vi "Get SLSC Module By Slot.vi"(8 "error in (no error)":errorcluster, 10 "Slot":i32, 11 "SLSC Chassis":u64) -> (0 "error out":errorcluster, 2 "SLSC Module":u64, 3 "SLSC Chassis out":u64)   [LabVIEW 2017, in "VeriStand SLSC Scripting.lvlib"]
uses:
  VeriStand SLSC Scripting.lvlib
  NationalInstruments.VeriStand.SystemDefinitionAPI
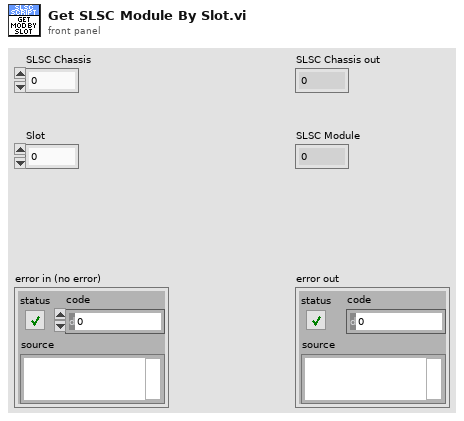
[diagram p1: front panel]
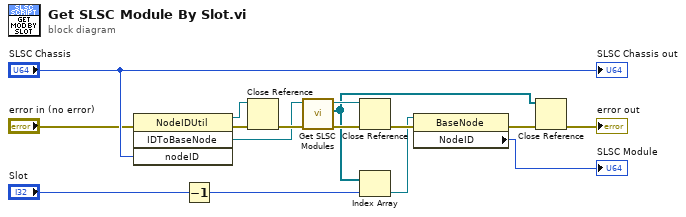
[diagram p0: block diagram]
diagram:
  n1 = invoke class="NodeIDUtil" method="IDToBaseNode"(error in="error in (no error)", "nodeID"="SLSC Chassis") -> (reference out=w15:refnum<k24>, error out=w16:errorcluster, "IDToBaseNode"=w13:refnum<k24>)  [unwired: 2 in, 1 out]
  n2 = Decrement(x="Slot") -> (x-1=w6:i32)
  n3 = Close Reference(reference=w15, error in (no error)=w16) -> (error out=w14:errorcluster)
  n4 = call "Get SLSC Modules.vi"("error in (no error)"=w14, "SLSC Chassis"=w13) -> ("error out"=w10:errorcluster, "SLSC Modules"=w2:refnum<k24>[], "SLSC Chassis out"=w8:refnum<k24>)  [unwired: 7 in]
  n5 = Close Reference(reference=w8, error in (no error)=w10) -> (error out=w9:errorcluster)
  n6 = Index Array(array=w2, index=w6) -> (element=w5:refnum<k24>)
  n7 = property class="BaseNode"(reference=w5, error in=w9) -> (error out=w4:errorcluster, "NodeID"=→"SLSC Module":u64)  [unwired: 1 out]
  n8 = Close Reference(reference=w2, error in (no error)=w4) -> (error out=→"error out":errorcluster)
  "SLSC Chassis out" <- "SLSC Chassis"
